vi "CustomErrorHandler.vi"() -> ()   [LabVIEW 2012]
panel:
  in  "Custom error description":string[](array[string])
  in  "Custom errors code":i32[](array[numeric])
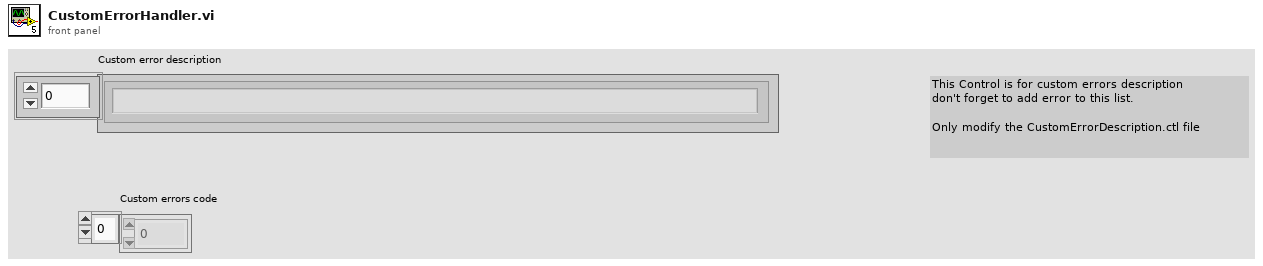
[diagram p1: front panel]
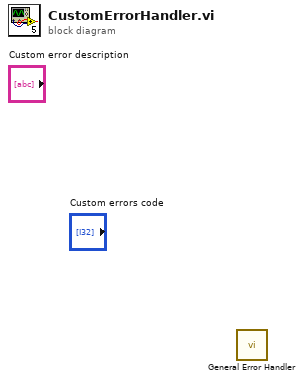
[diagram p0: block diagram]
diagram:
  n1 = call <vilib>:"General Error Handler.vi"() -> ()  [unwired: 11 in, 5 out]
